vi "IB_RW_Project_SoftDep.vi"(7 "action":T3, 8 "error in (no error)":errorcluster, 9 "index in":string, 10 "dataSource in":T2, 11 "buildObject":T1) -> (0 "error out":errorcluster, 1 "index out":string, 2 "dataSource out":T2, 3 "buildObject out":T1)   [LabVIEW 2020]
doc: "Reads and writes the data to the object property bag."
uses:
  <resource>/Framework/Providers/API/ItemRef.ctl
  <vilib>/AppBuilder/IB_RW_Project/IB_RW_Project_PropBag_Action.ctl
  <vilib>/AppBuilder/IB_RW_Project/IB_RW_Project_SoftDep_Data.ctl
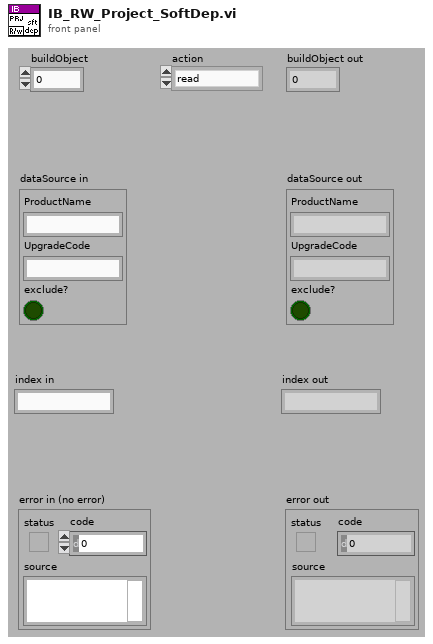
[diagram p1: front panel]
types:
  T1 = typedef "ItemRef.ctl" = u64
  T2 = typedef "IB_RW_Project_SoftDep_Data.ctl" = cluster{"ProductName":string, "UpgradeCode":string, "exclude?":bool}
  T3 = typedef "IB_RW_Project_PropBag_Action.ctl" = enum16{"read", "write", "clear", "readPrevious", "writePrevious", "clearPrevious"}
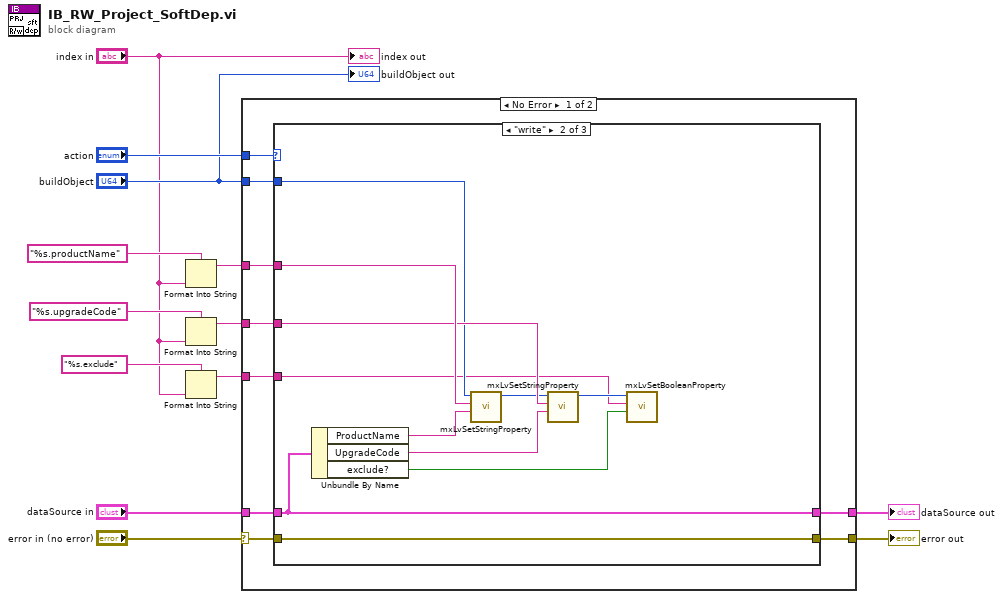
[diagram p0: block diagram]
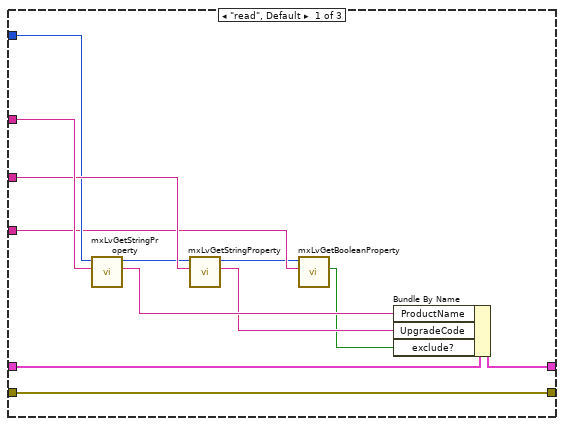
[diagram p2: hidden frame]
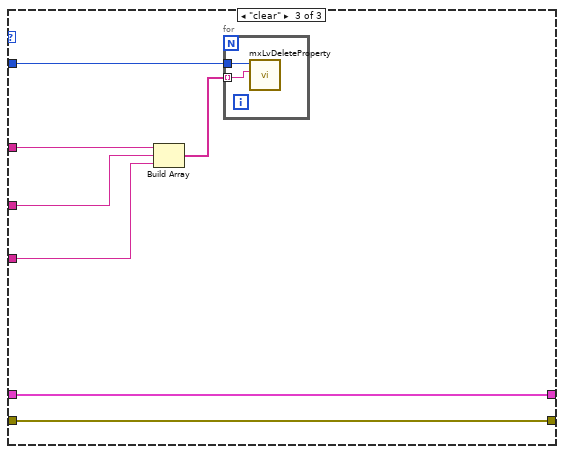
[diagram p3: hidden frame]
diagram:
  n1 = Format Into String(format string="%s.productName", "index in") -> (resulting string=w8:string)  [unwired: 2 in, 1 out]
  n2 = Format Into String(format string="%s.upgradeCode", "index in") -> (resulting string=w4:string)  [unwired: 2 in, 1 out]
  n3 = Format Into String(format string="%s.exclude", "index in") -> (resulting string=w1:string)  [unwired: 2 in, 1 out]
  n4 = case shown="No Error" "error in (no error)" {
    selector: "error in (no error)" -> [w18 w55]
    tunnel: "action" -> [w22 _]
    tunnel: "dataSource in" -> [w21 w56]
    tunnel: [w20 w56] -> w11
    tunnel: "buildObject" -> [w16 _]
    tunnel: w8 -> [w19 _]
    tunnel: [w15 w55] -> w7
    tunnel: w4 -> [w17 _]
    tunnel: w1 -> [w14 _]
    frame No Error {
      n5 = case shown="\"write\"" w22 {
        tunnel: w16 -> [w27 w39 w48]
        tunnel: w21 -> [w34 w45 w52]
        tunnel: [w33 w45 w52] -> w20
        tunnel: w19 -> [w32 w42 w50]
        tunnel: [w31 w44 w49] -> w15
        tunnel: w18 -> [w31 w44 w49]
        tunnel: w17 -> [w29 w41 w47]
        tunnel: w14 -> [w25 w35 w46]
        frame "read", Default {
          n6 = call <resource>:"mxLvGetStringProperty.vi"("Tag"=w32, "Item"=w27) -> ("Value"=w30:string, "Item"=w26:T1)  [unwired: 1 in, 7 out]
          n7 = call <resource>:"mxLvGetStringProperty.vi"("Tag"=w29, "Item"=w26) -> ("Value"=w28:string, "Item"=w24:T1)  [unwired: 1 in, 7 out]
          n8 = call <resource>:"mxLvGetBooleanProperty.vi"("Tag"=w25, "Item"=w24) -> ("Value"=w23:bool)  [unwired: 7 in, 2 out]
          n9 = Bundle By Name(cluster=w34, "ProductName"=w30, "UpgradeCode"=w28, "exclude?"=w23) -> (w33:T2)
        }
        frame "write" {
          n10 = Unbundle By Name(w45) -> ("ProductName"=w43:string, "UpgradeCode"=w40:string, "exclude?"=w36:bool)
          n11 = call <resource>:"mxLvSetStringProperty.vi"("Value (\"\")"=w43, "Tag"=w42, "Item"=w39) -> ("Item"=w38:T1)  [unwired: 2 in, 6 out]
          n12 = call <resource>:"mxLvSetStringProperty.vi"("Value (\"\")"=w40, "Tag"=w41, "Item"=w38) -> ("Item"=w37:T1)  [unwired: 2 in, 6 out]
          n13 = call <resource>:"mxLvSetBooleanProperty.vi"("Value (F)"=w36, "Tag"=w35, "Item"=w37) -> ()  [unwired: 7 in, 2 out]
        }
        frame "clear" {
          n14 = Build Array(w50, w47, w46) -> (w51:string[])
          n15 = for {
            tunnel: w51 -> [w54] mode=indexing
            tunnel: w48 -> [w53]
            n16 = call <resource>:"mxLvDeleteProperty.vi"("Tag"=w54, "Item"=w53) -> ()  [unwired: 1 in, 9 out]
          }
        }
      }
    }
    frame Error {
    }
  }
  "error out" <- w7
  "dataSource out" <- w11
  "buildObject out" <- "buildObject"
  "index out" <- "index in"
